vi "nanocal -- nuclear schottky fit V8.vi"() -> ()   [LabVIEW 2021] (continued)
 ,  \"στS\" -> 0.000000000000   ,  \"στN\" -> 0.000000000000   ,  \"τ11 \" -> 0.000000000000   ,  \"τ12\" -> 0.000000000000   ,  \"τ22\" -> 0.000000000000   ,  \"τN1\" -> 0.000000000000   ,  \"τN2\" -> 0.000000000000   ,  \"σηlogτ1 \" -> 0.000000000000   ,  \"σηlogτS\" -> 0.000000000000   ,  \"σηlogτN\" -> 0.000000000000   ,  \"σlogτ1\" -> 0.000000000000   ,  \"σlogτS\" -> 0.000000000000   ,  \"σlogτN\" -> 0.000000000000   ,  \"σητ1\" -> 0.000000000000   ,  \"σητS \" -> 0.000000000000   ,  \"σητN\" -> 0.000000000000    |>   , \r\"IDS0498_220603_RAW_cal__ref_\" ->   <|    \"ζ\" -> 0.110734162984   ,  \"τ1\" -> 0.019381596449   ,  \"τS\" -> 0.049800010244   ,  \"τN\" -> 0.007874153241   ,  \"τC\" -> 0.001094666009   ,  \"κ0\" -> 0.000000001580   ,  \"mm1\" -> 0.000107216591   ,  \"mm2\" -> 0.015930752272   ,  \"mm3\" -> 0.068498957299   ,  \"T\" -> 0.300000000000   ,  \"B\" -> 8.000000000000   ,  \"θ\" -> 45.000000000000   ,  \"Reoff\" -> -10657142.857142858200   ,  \"Imoff\" -> 0.000000000000   ,  \"στ1\" -> 0.007394501349   ,  \"στS\" -> 0.001744107422   ,  \"στN\" -> 0.001987690041   ,  \"τ11 \" -> 0.000000000000   ,  \"τ12\" -> 0.000000000000   ,  \"τ22\" -> 0.000000000000   ,  \"τN1\" -> 0.000000000000   ,  \"τN2\" -> 0.000000000000   ,  \"σηlogτ1 \" -> 0.000000000000   ,  \"σηlogτS\" -> 0.000000000000   ,  \"σηlogτN\" -> 0.000000000000   ,  \"σlogτ1\" -> 0.000000000000   ,  \"σlogτS\" -> 0.000000000000   ,  \"σlogτN\" -> 0.000000000000   ,  \"σητ1\" -> 0.000000000000   ,  \"σητS \" -> 0.000000000000   ,  \"σητN\" -> 0.000000000000    |>   , \r\"IDS0498_220603_RAW_cal__sam_\" ->   <|    \"ζ\" -> 0.000000000000   ,  \"τ1\" -> 0.000000000000   ,  \"τS\" -> 0.000000000000   ,  \"τN\" -> 0.000000000000   ,  \"τC\" -> 0.000000000000   ,  \"κ0\" -> 0.000000000000   ,  \"mm1\" -> 0.000000000000   ,  \"mm2\" -> 0.000000000000   ,  \"mm3\" -> 0.000000000000   ,  \"T\" -> 0.300000000000   ,  \"B\" -> 8.000000000000   ,  \"θ\" -> 45.000000000000   ,  \"Reoff\" -> 0.000000000000   ,  \"Imoff\" -> 0.000000000000   ,  \"στ1\" -> 0.000000000000   ,  \"στS\" -> 0.000000000000   ,  \"στN\" -> 0.000000000000   ,  \"τ11 \" -> 0.000000000000   ,  \"τ12\" -> 0.000000000000   ,  \"τ22\" -> 0.000000000000   ,  \"τN1\" -> 0.000000000000   ,  \"τN2\" -> 0.000000000000   ,  \"σηlogτ1 \" -> 0.000000000000   ,  \"σηlogτS\" -> 0.000000000000   ,  \"σηlogτN\" -> 0.000000000000   ,  \"σlogτ1\" -> 0.000000000000   ,  \"σlogτS\" -> 0.000000000000   ,  \"σlogτN\" -> 0.000000000000   ,  \"σητ1\" -> 0.000000000000   ,  \"σητS \" -> 0.000000000000   ,  \"σητN\" -> 0.000000000000    |>   , \r\"IDS0499_220603_RAW_cal__ref_\" ->   <|    \"ζ\" -> 0.075729964973   ,  \"τ1\" -> 0.017492157350   ,  \"τS\" -> 0.042916924435   ,  \"τN\" -> 0.003910009488   ,  \"τC\" -> 0.001485143735   ,  \"κ0\" -> 0.000000001996   ,  \"mm1\" -> 0.000101508308   ,  \"mm2\" -> 0.015465208626   ,  \"mm3\" -> 0.053783720140   ,  \"T\" -> 0.360000000000   ,  \"B\" -> 8.000000000000   ,  \"θ\" -> 45.000000000000   ,  \"Reoff\" -> -3787755.102040812380   ,  \"Imoff\" -> 0.000000000000   ,  \"στ1\" -> 0.001180089795   ,  \"στS\" -> 0.000447730504   ,  \"στN\" -> 0.000150733035   ,  \"τ11 \" -> 0.000000000000   ,  \"τ12\" -> 0.000000000000   ,  \"τ22\" -> 0.000000000000   ,  \"τN1\" -> 0.000000000000   ,  \"τN2\" -> 0.000000000000   ,  \"σηlogτ1 \" -> 0.000000000000   ,  \"σηlogτS\" -> 0.000000000000   ,  \"σηlogτN\" -> 0.000000000000   ,  \"σlogτ1\" -> 0.000000000000   ,  \"σlogτS\" -> 0.000000000000   ,  \"σlogτN\" -> 0.000000000000   ,  \"σητ1\" -> 0.000000000000   ,  \"σητS \" -> 0.000000000000   ,  \"σητN\" -> 0.000000000000    |>   , \r\"IDS0499_220603_RAW_cal__sam_\" ->   <|    \"ζ\" -> 0.000000000000   ,  \"τ1\" -> 0.000000000000   ,  \"τS\" -> 0.000000000000   ,  \"τN\" -> 0.000000000000   ,  \"τC\" -> 0.000000000000   ,  \"κ0\" -> 0.000000000000   ,  \"mm1\" -> 0.000000000000   ,  \"mm2\" -> 0.000000000000   ,  \"mm3\" -> 0.000000000000   ,  \"T\" -> 0.360000000000   ,  \"B\" -> 8.000000000000   ,  \"θ\" -> 45.000000000000   ,  \"Reoff\" -> 0.000000000000   ,  \"Imoff\" -> 0.000000000000   ,  \"στ1\" -> 0.000000000000   ,  \"στS\" -> 0.000000000000   ,  \"στN\" -> 0.000000000000   ,  \"τ11 \" -> 0.000000000000   ,  \"τ12\" -> 0.000000000000   ,  \"τ22\" -> 0.000000000000   ,  \"τN1\" -> 0.000000000000   ,  \"τN2\" -> 0.000000000000   ,  \"σηlogτ1 \" -> 0.000000000000   ,  \"σηlogτS\" -> 0.000000000000   ,  \"σηlogτN\" -> 0.000000000000   ,  \"σlogτ1\" -> 0.000000000000   ,  \"σlogτS\" -> 0.000000000000   ,  \"σlogτN\" -> 0.000000000000   ,  \"σητ1\" -> 0.000000000000   ,  \"σητS \" -> 0.000000000000   ,  \"σητN\" -> 0.000000000000    |>   , \r\"IDS0500_220603_RAW_cal__ref_\" ->   <|    \"ζ\" -> 0.057062025730   ,  \"τ1\" -> 0.015621328716   ,  \"τS\" -> 0.037684759429   ,  \"τN\" -> 0.002528358408   ,  \"τC\" -> 0.001814587656   ,  \"κ0\" -> 0.000000002409   ,  \"mm1\" -> 0.000093897005   ,  \"mm2\" -> 0.014229954054   ,  \"mm3\" -> 0.045619825114   ,  \"T\" -> 0.420000000000   ,  \"B\" -> 8.000000000000   ,  \"θ\" -> 45.000000000000   ,  \"Reoff\" -> -1914285.714285716420   ,  \"Imoff\" -> 0.000000000000   ,  \"στ1\" -> 0.000955516526   ,  \"στS\" -> 0.000234895501   ,  \"στN\" -> 0.000135281330   ,  \"τ11 \" -> 0.000000000000   ,  \"τ12\" -> 0.000000000000   ,  \"τ22\" -> 0.000000000000   ,  \"τN1\" -> 0.000000000000   ,  \"τN2\" -> 0.000000000000   ,  \"σηlogτ1 \" -> 0.000000000000   ,  \"σηlogτS\" -> 0.000000000000   ,  \"σηlogτN\" -> 0.000000000000   ,  \"σlogτ1\" -> 0.000000000000   ,  \"σlogτS\" -> 0.000000000000   ,  \"σlogτN\" -> 0.000000000000   ,  \"σητ1\" -> 0.000000000000   ,  \"σητS \" -> 0.000000000000   ,  \"σητN\" -> 0.000000000000    |>   , \r\"IDS0500_220603_RAW_cal__sam_\" ->   <|    \"ζ\" -> 0.000000000000   ,  \"τ1\" -> 0.000000000000   ,  \"τS\" -> 0.000000000000   ,  \"τN\" -> 0.000000000000   ,  \"τC\" -> 0.000000000000   ,  \"κ0\" -> 0.000000000000   ,  \"mm1\" -> 0.000000000000   ,  \"mm2\" -> 0.000000000000   ,  \"mm3\" -> 0.000000000000   ,  \"T\" -> 0.420000000000   ,  \"B\" -> 8.000000000000   ,  \"θ\" -> 45.000000000000   ,  \"Reoff\" -> 0.000000000000   ,  \"Imoff\" -> 0.000000000000   ,  \"στ1\" -> 0.000000000000   ,  \"στS\" -> 0.000000000000   ,  \"στN\" -> 0.000000000000   ,  \"τ11 \" -> 0.000000000000   ,  \"τ12\" -> 0.000000000000   ,  \"τ22\" -> 0.000000000000   ,  \"τN1\" -> 0.000000000000   ,  \"τN2\" -> 0.000000000000   ,  \"σηlogτ1 \" -> 0.000000000000   ,  \"σηlogτS\" -> 0.000000000000   ,  \"σηlogτN\" -> 0.000000000000   ,  \"σlogτ1\" -> 0.000000000000   ,  \"σlogτS\" -> 0.000000000000   ,  \"σlogτN\" -> 0.000000000000   ,  \"σητ1\" -> 0.000000000000   ,  \"σητS \" -> 0.000000000000   ,  \"σητN\" -> 0.000000000000    |>   , \r\"IDS0501_220603_RAW_cal__ref_\" ->   <|    \"ζ\" -> 0.041820610943   ,  \"τ1\" -> 0.014727705147   ,  \"τS\" -> 0.032103066270   ,  \"τN\" -> 0.001402697929   ,  \"τC\" -> 0.002062288671   ,  \"κ0\" -> 0.000000003070   ,  \"mm1\" -> 0.000078146988   ,  \"mm2\" -> 0.013796091461   ,  \"mm3\" -> 0.037822751096   ,  \"T\" -> 0.520000000000   ,  \"B\" -> 8.000000000000   ,  \"θ\" -> 45.000000000000   ,  \"Reoff\" -> -1155102.040816326160   ,  \"Imoff\" -> 0.000000000000   ,  \"στ1\" -> 0.000294282186   ,  \"στS\" -> 0.000104705305   ,  \"στN\" -> 0.000024302938   ,  \"τ11 \" -> 0.000000000000   ,  \"τ12\" -> 0.000000000000   ,  \"τ22\" -> 0.000000000000   ,  \"τN1\" -> 0.000000000000   ,  \"τN2\" -> 0.000000000000   ,  \"σηlogτ1 \" -> 0.000000000000   ,  \"σηlogτS\" -> 0.000000000000   ,  \"σηlogτN\" -> 0.000000000000   ,  \"σlogτ1\" -> 0.000000000000   ,  \"σlogτS\" -> 0.000000000000   ,  \"σlogτN\" -> 0.000000000000   ,  \"σητ1\" -> 0.000000000000   ,  \"σητS \" -> 0.000000000000   ,  \"σητN\" -> 0.000000000000    |>   , \r\"IDS0501_220603_RAW_cal__sam_\" ->   <|    \"ζ\" -> 0.000000000000   ,  \"τ1\" -> 0.000000000000   ,  \"τS\" -> 0.000000000000   ,  \"τN\" -> 0.000000000000   ,  \"τC\" -> 0.000000000000   ,  \"κ0\" -> 0.000000000000   ,  \"mm1\" -> 0.000000000000   ,  \"mm2\" -> 0.000000000000   ,  \"mm3\" -> 0.000000000000   ,  \"T\" -> 0.520000000000   ,  \"B\" -> 8.000000000000   ,  \"θ\" -> 45.000000000000   ,  \"Reoff\" -> 0.000000000000   ,  \"Imoff\" -> 0.000000000000   ,  \"στ1\" -> 0.000000000000   ,  \"στS\" -> 0.000000000000   ,  \"στN\" -> 0.000000000000   ,  \"τ11 \" -> 0.000000000000   ,  \"τ12\" -> 0.000000000000   ,  \"τ22\" -> 0.000000000000   ,  \"τN1\" -> 0.000000000000   ,  \"τN2\" -> 0.000000000000   ,  \"σηlogτ1 \" -> 0.000000000000   ,  \"σηlogτS\" -> 0.000000000000   ,  \"σηlogτN\" -> 0.000000000000   ,  \"σlogτ1\" -> 0.000000000000   ,  \"σlogτS\" -> 0.000000000000   ,  \"σlogτN\" -> 0.000000000000   ,  \"σητ1\" -> 0.000000000000   ,  \"σητS \" -> 0.000000000000   ,  \"σητN\" -> 0.000000000000    |>   , \r\"IDS0502_220603_RAW_cal__ref_\" ->   <|    \"ζ\" -> 0.034670986979   ,  \"τ1\" -> 0.014178027620   ,  \"τS\" -> 0.028243061757   ,  \"τN\" -> 0.000956770293   ,  \"τC\" -> 0.002118106957   ,  \"κ0\" -> 0.000000003766   ,  \"mm1\" -> 0.000066318852   ,  \"mm2\" -> 0.013432939767   ,  \"mm3\" -> 0.033009095005   ,  \"T\" -> 0.620000000000   ,  \"B\" -> 8.000000000000   ,  \"θ\" -> 45.000000000000   ,  \"Reoff\" -> -1228571.428571428170   ,  \"Imoff\" -> 0.000000000000   ,  \"στ1\" -> 0.000460475840   ,  \"στS\" -> 0.000103102463   ,  \"στN\" -> 0.000021520778   ,  \"τ11 \" -> 0.000000000000   ,  \"τ12\" -> 0.000000000000   ,  \"τ22\" -> 0.000000000000   ,  \"τN1\" -> 0.000000000000   ,  \"τN2\" -> 0.000000000000   ,  \"σηlogτ1 \" -> 0.000000000000   ,  \"σηlogτS\" -> 0.000000000000   ,  \"σηlogτN\" -> 0.000000000000   ,  \"σlogτ1\" -> 0.000000000000   ,  \"σlogτS\" -> 0.000000000000   ,  \"σlogτN\" -> 0.000000000000   ,  \"σητ1\" -> 0.000000000000   ,  \"σητS \" -> 0.000000000000   ,  \"σητN\" -> 0.000000000000    |>   , \r\"IDS0502_220603_RAW_cal__sam_\" ->   <|    \"ζ\" -> 0.000000000000   ,  \"τ1\" -> 0.000000000000   ,  \"τS\" -> 0.000000000000   ,  \"τN\" -> 0.000000000000   ,  \"τC\" -> 0.000000000000   ,  \"κ0\" -> 0.000000000000   ,  \"mm1\" -> 0.000000000000   ,  \"mm2\" -> 0.000000000000   ,  \"mm3\" -> 0.000000000000   ,  \"T\" -> 0.620000000000   ,  \"B\" -> 8.000000000000   ,  \"θ\" -> 45.000000000000   ,  \"Reoff\" -> 0.000000000000   ,  \"Imoff\" -> 0.000000000000   ,  \"στ1\" -> 0.000000000000   ,  \"στS\" -> 0.000000000000   ,  \"στN\" -> 0.000000000000   ,  \"τ11 \" -> 0.000000000000   ,  \"τ12\" -> 0.000000000000   ,  \"τ22\" -> 0.000000000000   ,  \"τN1\" -> 0.000000000000   ,  \"τN2\" -> 0.000000000000   ,  \"σηlogτ1 \" -> 0.000000000000   ,  \"σηlogτS\" -> 0.000000000000   ,  \"σηlogτN\" -> 0.000000000000   ,  \"σlogτ1\" -> 0.000000000000   ,  \"σlogτS\" -> 0.000000000000   ,  \"σlogτN\" -> 0.000000000000   ,  \"σητ1\" -> 0.000000000000   ,  \"σητS \" -> 0.000000000000   ,  \"σητN\" -> 0.000000000000    |>   , \r\"IDS0503_220603_RAW_cal__ref_\" ->   <|    \"ζ\" -> 0.027095379561   ,  \"τ1\" -> 0.013653054815   ,  \"τS\" -> 0.022995805893   ,  \"τN\" -> 0.000345510729   ,  \"τC\" -> 0.002402226581   ,  \"κ0\" -> 0.000000005139   ,  \"mm1\" -> 0.000057649125   ,  \"mm2\" -> 0.013281563049   ,  \"mm3\" -> 0.026689827678   ,  \"T\" -> 0.820000000000   ,  \"B\" -> 8.000000000000   ,  \"θ\" -> 45.000000000000   ,  \"Reoff\" -> -959183.673469387459   ,  \"Imoff\" -> 0.000000000000   ,  \"στ1\" -> 0.008451198848   ,  \"στS\" -> 0.000084348723   ,  \"στN\" -> 0.004631417027   ,  \"τ11 \" -> 0.000000000000   ,  \"τ12\" -> 0.000000000000   ,  \"τ22\" -> 0.000000000000   ,  \"τN1\" -> 0.000000000000   ,  \"τN2\" -> 0.000000000000   ,  \"σηlogτ1 \" -> 0.000000000000   ,  \"σηlogτS\" -> 0.000000000000   ,  \"σηlogτN\" -> 0.000000000000   ,  \"σlogτ1\" -> 0.000000000000   ,  \"σlogτS\" -> 0.000000000000   ,  \"σlogτN\" -> 0.000000000000   ,  \"σητ1\" -> 0.000000000000   ,  \"σητS \" -> 0.000000000000   ,  \"σητN\" -> 0.000000000000    |>   , \r\"IDS0503_220603_RAW_cal__sam_\" ->   <|    \"ζ\" -> 0.000000000000   ,  \"τ1\" -> 0.000000000000   ,  \"τS\" -> 0.000000000000   ,  \"τN\" -> 0.000000000000   ,  \"τC\" -> 0.000000000000   ,  \"κ0\" -> 0.000000000000   ,  \"mm1\" -> 0.000000000000   ,  \"mm2\" -> 0.000000000000   ,  \"mm3\" -> 0.000000000000   ,  \"T\" -> 0.820000000000   ,  \"B\" -> 8.000000000000   ,  \"θ\" -> 45.000000000000   ,  \"Reoff\" -> 0.000000000000   ,  \"Imoff\" -> 0.000000000000   ,  \"στ1\" -> 0.000000000000   ,  \"στS\" -> 0.000000000000   ,  \"στN\" -> 0.000000000000   ,  \"τ11 \" -> 0.000000000000   ,  \"τ12\" -> 0.000000000000   ,  \"τ22\" -> 0.000000000000   ,  \"τN1\" -> 0.000000000000   ,  \"τN2\" -> 0.000000000000   ,  \"σηlogτ1 \" -> 0.000000000000   ,  \"σηlogτS\" -> 0.000000000000   ,  \"σηlogτN\" -> 0.000000000000   ,  \"σlogτ1\" -> 0.000000000000   ,  \"σlogτS\" -> 0.000000000000   ,  \"σlogτN\" -> 0.000000000000   ,  \"σητ1\" -> 0.000000000000   ,  \"σητS \" -> 0.000000000000   ,  \"σητN\" -> 0.000000000000    |>   , \r\"IDS0504_220603_RAW_cal__ref_\" ->   <|    \"ζ\" -> 0.022447798358   ,  \"τ1\" -> 0.013732237823   ,  \"τS\" -> 0.018577417913   ,  \"τN\" -> 0.000137993980   ,  \"τC\" -> 0.002459582749   ,  \"κ0\" -> 0.000000007201   ,  \"mm1\" -> 0.000047916113   ,  \"mm2\" -> 0.013491821681   ,  \"mm3\" -> 0.021787614463   ,  \"T\" -> 1.120000000000   ,  \"B\" -> 8.000000000000   ,  \"θ\" -> 45.000000000000   ,  \"Reoff\" -> -714285.714285713619   ,  \"Imoff\" -> 0.000000000000   ,  \"στ1\" -> 0.022424406509   ,  \"στS\" -> 0.000101728053   ,  \"στN\" -> 0.011081871918   ,  \"τ11 \" -> 0.000000000000   ,  \"τ12\" -> 0.000000000000   ,  \"τ22\" -> 0.000000000000   ,  \"τN1\" -> 0.000000000000   ,  \"τN2\" -> 0.000000000000   ,  \"σηlogτ1 \" -> 0.000000000000   ,  \"σηlogτS\" -> 0.000000000000   ,  \"σηlogτN\" -> 0.000000000000   ,  \"σlogτ1\" -> 0.000000000000   ,  \"σlogτS\" -> 0.000000000000   ,  \"σlogτN\" -> 0.000000000000   ,  \"σητ1\" -> 0.000000000000   ,  \"σητS \" -> 0.000000000000   ,  \"σητN\" -> 0.000000000000    |>   , \r\"IDS0504_220603_RAW_cal__sam_\" ->   <|    \"ζ\" -> 0.000000000000   ,  \"τ1\" -> 0.000000000000   ,  \"τS\" -> 0.000000000000   ,  \"τN\" -> 0.000000000000   ,  \"τC\" -> 0.000000000000   ,  \"κ0\" -> 0.000000000000   ,  \"mm1\" -> 0.000000000000   ,  \"mm2\" -> 0.000000000000   ,  \"mm3\" -> 0.000000000000   ,  \"T\" -> 1.120000000000   ,  \"B\" -> 8.000000000000   ,  \"θ\" -> 45.000000000000   ,  \"Reoff\" -> 0.000000000000   ,  \"Imoff\" -> 0.000000000000   ,  \"στ1\" -> 0.000000000000   ,  \"στS\" -> 0.000000000000   ,  \"στN\" -> 0.000000000000   ,  \"τ11 \" -> 0.000000000000   ,  \"τ12\" -> 0.000000000000   ,  \"τ22\" -> 0.000000000000   ,  \"τN1\" -> 0.000000000000   ,  \"τN2\" -> 0.000000000000   ,  \"σηlogτ1 \" -> 0.000000000000   ,  \"σηlogτS\" -> 0.000000000000   ,  \"σηlogτN\" -> 0.000000000000   ,  \"σlogτ1\" -> 0.000000000000   ,  \"σlogτS\" -> 0.000000000000   ,  \"σlogτN\" -> 0.000000000000   ,  \"σητ1\" -> 0.000000000000   ,  \"σητS \" -> 0.000000000000   ,  \"σητN\" -> 0.000000000000    |>   , \r\"IDS0505_220603_RAW_cal__ref_\" ->   <|    \"ζ\" -> 0.017603951649   ,  \"τ1\" -> 0.013742471601   ,  \"τS\" -> 0.012869162108   ,  \"τN\" -> 0.000030445804   ,  \"τC\" -> 0.002783258647   ,  \"κ0\" -> 0.000000012669   ,  \"mm1\" -> 0.000039809007   ,  \"mm2\" -> 0.013558407618   ,  \"mm3\" -> 0.016054205609   ,  \"T\" -> 1.900000000000   ,  \"B\" -> 8.000000000000   ,  \"θ\" -> 45.000000000000   ,  \"Reoff\" -> -322448.979591836221   ,  \"Imoff\" -> 0.000000000000   ,  \"στ1\" -> 0.123558852950   ,  \"στS\" -> 0.000153637870   ,  \"στN\" -> 0.054392603462   ,  \"τ11 \" -> 0.000000000000   ,  \"τ12\" -> 0.000000000000   ,  \"τ22\" -> 0.000000000000   ,  \"τN1\" -> 0.000000000000   ,  \"τN2\" -> 0.000000000000   ,  \"σηlogτ1 \" -> 0.000000000000   ,  \"σηlogτS\" -> 0.000000000000   ,  \"σηlogτN\" -> 0.000000000000   ,  \"σlogτ1\" -> 0.000000000000   ,  \"σlogτS\" -> 0.000000000000   ,  \"σlogτN\" -> 0.000000000000   ,  \"σητ1\" -> 0.000000000000   ,  \"σητS \" -> 0.000000000000   ,  \"σητN\" -> 0.000000000000    |>   , \r\"IDS0505_220603_RAW_cal__sam_\" ->   <|    \"ζ\" -> 0.000000000000   ,  \"τ1\" -> 0.000000000000   ,  \"τS\" -> 0.000000000000   ,  \"τN\" -> 0.000000000000   ,  \"τC\" -> 0.000000000000   ,  \"κ0\" -> 0.000000000000   ,  \"mm1\" -> 0.000000000000   ,  \"mm2\" -> 0.000000000000   ,  \"mm3\" -> 0.000000000000   ,  \"T\" -> 1.900000000000   ,  \"B\" -> 8.000000000000   ,  \"θ\" -> 45.000000000000   ,  \"Reoff\" -> 0.000000000000   ,  \"Imoff\" -> 0.000000000000   ,  \"στ1\" -> 0.000000000000   ,  \"στS\" -> 0.000000000000   ,  \"στN\" -> 0.000000000000   ,  \"τ11 \" -> 0.000000000000   ,  \"τ12\" -> 0.000000000000   ,  \"τ22\" -> 0.000000000000   ,  \"τN1\" -> 0.000000000000   ,  \"τN2\" -> 0.000000000000   ,  \"σηlogτ1 \" -> 0.000000000000   ,  \"σηlogτS\" -> 0.000000000000   ,  \"σηlogτN\" -> 0.000000000000   ,  \"σlogτ1\" -> 0.000000000000   ,  \"σlogτS\" -> 0.000000000000   ,  \"σlogτN\" -> 0.000000000000   ,  \"σητ1\" -> 0.000000000000   ,  \"σητS \" -> 0.000000000000   ,  \"σητN\" -> 0.000000000000    |>   , \r\"IDS0506_220603_RAW_cal__ref_\" ->   <|    \"ζ\" -> 0.017513535650   ,  \"τ1\" -> 0.013742433942   ,  \"τS\" -> 0.009294247030   ,  \"τN\" -> 0.000005722768   ,  \"τC\" -> 0.002563999230   ,  \"κ0\" -> 0.000000022469   ,  \"mm1\" -> 0.000034819634   ,  \"mm2\" -> 0.011947473488   ,  \"mm3\" -> 0.013786985200   ,  \"T\" -> 3.100000000000   ,  \"B\" -> 8.000000000000   ,  \"θ\" -> 45.000000000000   ,  \"Reoff\" -> -175510.204081632197   ,  \"Imoff\" -> 0.000000000000   ,  \"στ1\" -> 0.880762480846   ,  \"στS\" -> 0.000241080362   ,  \"στN\" -> 0.387161662293   ,  \"τ11 \" -> 0.000000000000   ,  \"τ12\" -> 0.000000000000   ,  \"τ22\" -> 0.000000000000   ,  \"τN1\" -> 0.000000000000   ,  \"τN2\" -> 0.000000000000   ,  \"σηlogτ1 \" -> 0.000000000000   ,  \"σηlogτS\" -> 0.000000000000   ,  \"σηlogτN\" -> 0.000000000000   ,  \"σlogτ1\" -> 0.000000000000   ,  \"σlogτS\" -> 0.000000000000   ,  \"σlogτN\" -> 0.000000000000   ,  \"σητ1\" -> 0.000000000000   ,  \"σητS \" -> 0.000000000000   ,  \"σητN\" -> 0.000000000000    |>   , \r\"IDS0506_220603_RAW_cal__sam_\" ->   <|    \"ζ\" -> 0.000000000000   ,  \"τ1\" -> 0.000000000000   ,  \"τS\" -> 0.000000000000   ,  \"τN\" -> 0.000000000000   ,  \"τC\" -> 0.000000000000   ,  \"κ0\" -> 0.000000000000   ,  \"mm1\" -> 0.000000000000   ,  \"mm2\" -> 0.000000000000   ,  \"mm3\" -> 0.000000000000   ,  \"T\" -> 3.100000000000   ,  \"B\" -> 8.000000000000   ,  \"θ\" -> 45.000000000000   ,  \"Reoff\" -> 0.000000000000   ,  \"Imoff\" -> 0.000000000000   ,  \"στ1\" -> 0.000000000000   ,  \"στS\" -> 0.000000000000   ,  \"στN\" -> 0.000000000000   ,  \"τ11 \" -> 0.000000000000   ,  \"τ12\" -> 0.000000000000   ,  \"τ22\" -> 0.000000000000   ,  \"τN1\" -> 0.000000000000   ,  \"τN2\" -> 0.000000000000   ,  \"σηlogτ1 \" -> 0.000000000000   ,  \"σηlogτS\" -> 0.000000000000   ,  \"σηlogτN\" -> 0.000000000000   ,  \"σlogτ1\" -> 0.000000000000   ,  \"σlogτS\" -> 0.000000000000   ,  \"σlogτN\" -> 0.000000000000   ,  \"σητ1\" -> 0.000000000000   ,  \"σητS \" -> 0.000000000000   ,  \"σητN\" -> 0.000000000000    |>   , \r\"IDS0508_220603_RAW_cal__ref_\" ->   <|    \"ζ\" -> 0.243281471751   ,  \"τ1\" -> 0.025048654847   ,  \"τS\" -> 0.062611130643   ,  \"τN\" -> 0.020042988527   ,  \"τC\" -> 0.000849297815   ,  \"κ0\" -> 0.000000000907   ,  \"mm1\" -> 0.000164736185   ,  \"mm2\" -> 0.017764187201   ,  \"mm3\" -> 0.110731364203   ,  \"T\" -> 0.200000000000   ,  \"B\" -> 6.000000000000   ,  \"θ\" -> 45.000000000000   ,  \"Reoff\" -> -40636734.693877548000   ,  \"Imoff\" -> 0.000000000000   ,  \"στ1\" -> 0.014234353727   ,  \"στS\" -> 0.004838976210   ,  \"στN\" -> 0.004976250052   ,  \"τ11 \" -> 0.000000000000   ,  \"τ12\" -> 0.000000000000   ,  \"τ22\" -> 0.000000000000   ,  \"τN1\" -> 0.000000000000   ,  \"τN2\" -> 0.000000000000   ,  \"σηlogτ1 \" -> 0.000000000000   ,  \"σηlogτS\" -> 0.000000000000   ,  \"σηlogτN\" -> 0.000000000000   ,  \"σlogτ1\" -> 0.000000000000   ,  \"σlogτS\" -> 0.000000000000   ,  \"σlogτN\" -> 0.000000000000   ,  \"σητ1\" -> 0.000000000000   ,  \"σητS \" -> 0.000000000000   ,  \"σητN\" -> 0.000000000000    |>   , \r\"IDS0508_220603_RAW_cal__sam_\" ->   <|    \"ζ\" -> 0.000000000000   ,  \"τ1\" -> 0.000000000000   ,  \"τS\" -> 0.000000000000   ,  \"τN\" -> 0.000000000000   ,  \"τC\" -> 0.000000000000   ,  \"κ0\" -> 0.000000000000   ,  \"mm1\" -> 0.000000000000   ,  \"mm2\" -> 0.000000000000   ,  \"mm3\" -> 0.000000000000   ,  \"T\" -> 0.200000000000   ,  \"B\" -> 6.000000000000   ,  \"θ\" -> 45.000000000000   ,  \"Reoff\" -> 0.000000000000   ,  \"Imoff\" -> 0.000000000000   ,  \"στ1\" -> 0.000000000000   ,  \"στS\" -> 0.000000000000   ,  \"στN\" -> 0.000000000000   ,  \"τ11 \" -> 0.000000000000   ,  \"τ12\" -> 0.000000000000   ,  \"τ22\" -> 0.000000000000   ,  \"τN1\" -> 0.000000000000   ,  \"τN2\" -> 0.000000000000   ,  \"σηlogτ1 \" -> 0.000000000000   ,  \"σηlogτS\" -> 0.000000000000   ,  \"σηlogτN\" -> 0.000000000000   ,  \"σlogτ1\" -> 0.000000000000   ,  \"σlogτS\" -> 0.000000000000   ,  \"σlogτN\" -> 0.000000000000   ,  \"σητ1\" -> 0.000000000000   ,  \"σητS \" -> 0.000000000000   ,  \"σητN\" -> 0.000000000000    |>   , \r\"IDS0509_220603_RAW_cal__ref_\" ->   <|    \"ζ\" -> 0.413507557358   ,  \"τ1\" -> 0.033675995603   ,  \"τS\" -> 0.093816108912   ,  \"τN\" -> 0.061390510422   ,  \"τC\" -> 0.000803159189   ,  \"κ0\" -> 0.000000000612   ,  \"mm1\" -> 0.000233947412   ,  \"mm2\" -> 0.019125451380   ,  \"mm3\" -> 0.234505485381   ,  \"T\" -> 0.150000000000   ,  \"B\" -> 6.000000000000   ,  \"θ\" -> 45.000000000000   ,  \"Reoff\" -> -88975510.204081654600   ,  \"Imoff\" -> 0.000000000000   ,  \"στ1\" -> 0.030359635336   ,  \"στS\" -> 0.022777334435   ,  \"στN\" -> 0.025753606266   ,  \"τ11 \" -> 0.000000000000   ,  \"τ12\" -> 0.000000000000   ,  \"τ22\" -> 0.000000000000   ,  \"τN1\" -> 0.000000000000   ,  \"τN2\" -> 0.000000000000   ,  \"σηlogτ1 \" -> 0.000000000000   ,  \"σηlogτS\" -> 0.000000000000   ,  \"σηlogτN\" -> 0.000000000000   ,  \"σlogτ1\" -> 0.000000000000   ,  \"σlogτS\" -> 0.000000000000   ,  \"σlogτN\" -> 0.000000000000   ,  \"σητ1\" -> 0.000000000000   ,  \"σητS \" -> 0.000000000000   ,  \"σητN\" -> 0.000000000000    |>   , \r\"IDS0509_220603_RAW_cal__sam_\" ->   <|    \"ζ\" -> 0.000000000000   ,  \"τ1\" -> 0.000000000000   ,  \"τS\" -> 0.000000000000   ,  \"τN\" -> 0.000000000000   ,  \"τC\" -> 0.000000000000   ,  \"κ0\" -> 0.000000000000   ,  \"mm1\" -> 0.000000000000   ,  \"mm2\" -> 0.000000000000   ,  \"mm3\" -> 0.000000000000   ,  \"T\" -> 0.150000000000   ,  \"B\" -> 6.000000000000   ,  \"θ\" -> 45.000000000000   ,  \"Reoff\" -> 0.000000000000   ,  \"Imoff\" -> 0.000000000000   ,  \"στ1\" -> 0.000000000000   ,  \"στS\" -> 0.000000000000   ,  \"στN\" -> 0.000000000000   ,  \"τ11 \" -> 0.000000000000   ,  \"τ12\" -> 0.000000000000   ,  \"τ22\" -> 0.000000000000   ,  \"τN1\" -> 0.000000000000   ,  \"τN2\" -> 0.000000000000   ,  \"σηlogτ1 \" -> 0.000000000000   ,  \"σηlogτS\" -> 0.000000000000   ,  \"σηlogτN\" -> 0.000000000000   ,  \"σlogτ1\" -> 0.000000000000   ,  \"σlogτS\" -> 0.000000000000   ,  \"σlogτN\" -> 0.000000000000   ,  \"σητ1\" -> 0.000000000000   ,  \"σητS \" -> 0.000000000000   ,  \"σητN\" -> 0.000000000000    |>   , \r\"IDS0510_220603_RAW_cal__ref_\" ->   <|    \"ζ\" -> 0.613284276562   ,  \"τ1\" -> 0.039588841090   ,  \"τS\" -> 0.126363579952   ,  \"τN\" -> 0.150529821612   ,  \"τC\" -> 0.000834158039   ,  \"κ0\" -> 0.000000000449   ,  \"mm1\" -> 0.000316290952   ,  \"mm2\" -> 0.017230786632   ,  \"mm3\" -> 0.469583692571   ,  \"T\" -> 0.120000000000   ,  \"B\" -> 6.000000000000   ,  \"θ\" -> 45.000000000000   ,  \"Reoff\" -> -183040816.326530635000   ,  \"Imoff\" -> 0.000000000000   ,  \"στ1\" -> 0.058972518993   ,  \"στS\" -> 0.069910296081   ,  \"στN\" -> 0.097464298744   ,  \"τ11 \" -> 0.000000000000   ,  \"τ12\" -> 0.000000000000   ,  \"τ22\" -> 0.000000000000   ,  \"τN1\" -> 0.000000000000   ,  \"τN2\" -> 0.000000000000   ,  \"σηlogτ1 \" -> 0.000000000000   ,  \"σηlogτS\" -> 0.000000000000   ,  \"σηlogτN\" -> 0.000000000000   ,  \"σlogτ1\" -> 0.000000000000   ,  \"σlogτS\" -> 0.000000000000   ,  \"σlogτN\" -> 0.000000000000   ,  \"σητ1\" -> 0.000000000000   ,  \"σητS \" -> 0.000000000000   ,  \"σητN\" -> 0.000000000000    |>   , \r\"IDS0510_220603_RAW_cal__sam_\" ->   <|    \"ζ\" -> 0.000000000000   ,  \"τ1\" -> 0.000000000000   ,  \"τS\" -> 0.000000000000   ,  \"τN\" -> 0.000000000000   ,  \"τC\" -> 0.000000000000   ,  \"κ0\" -> 0.000000000000   ,  \"mm1\" -> 0.000000000000   ,  \"mm2\" -> 0.000000000000   ,  \"mm3\" -> 0.000000000000   ,  \"T\" -> 0.120000000000   ,  \"B\" -> 6.000000000000   ,  \"θ\" -> 45.000000000000   ,  \"Reoff\" -> 0.000000000000   ,  \"Imoff\" -> 0.000000000000   ,  \"στ1\" -> 0.000000000000   ,  \"στS\" -> 0.000000000000   ,  \"στN\" -> 0.000000000000   ,  \"τ11 \" -> 0.000000000000   ,  \"τ12\" -> 0.000000000000   ,  \"τ22\" -> 0.000000000000   ,  \"τN1\" -> 0.000000000000   ,  \"τN2\" -> 0.000000000000   ,  \"σηlogτ1 \" -> 0.000000000000   ,  \"σηlogτS\" -> 0.000000000000   ,  \"σηlogτN\" -> 0.000000000000   ,  \"σlogτ1\" -> 0.000000000000   ,  \"σlogτS\" -> 0.000000000000   ,  \"σlogτN\" -> 0.000000000000   ,  \"σητ1\" -> 0.000000000000   ,  \"σητS \" -> 0.000000000000   ,  \"σητN\" -> 0.000000000000    |>   , \r\"IDS0511_220604_RAW_cal__ref_\" ->   <|    \"ζ\" -> 0.330310083388   ,  \"τ1\" -> 0.030298910704   ,  \"τS\" -> 0.075236256272   ,  \"τN\" -> 0.040258490760   ,  \"τC\" -> 0.000782924983   ,  \"κ0\" -> 0.000000000728   ,  \"mm1\" -> 0.000193254303   ,  \"mm2\" -> 0.018356930637   ,  \"mm3\" -> 0.166175477301   ,  \"T\" -> 0.170000000000   ,  \"B\" -> 6.000000000000   ,  \"θ\" -> 45.000000000000   ,  \"Reoff\" -> -64436734.693877577800   ,  \"Imoff\" -> 0.000000000000   ,  \"στ1\" -> 0.014626951982   ,  \"στS\" -> 0.008056203133   ,  \"στN\" -> 0.008938953770   ,  \"τ11 \" -> 0.000000000000   ,  \"τ12\" -> 0.000000000000   ,  \"τ22\" -> 0.000000000000   ,  \"τN1\" -> 0.000000000000   ,  \"τN2\" -> 0.000000000000   ,  \"σηlogτ1 \" -> 0.000000000000   ,  \"σηlogτS\" -> 0.000000000000   ,  \"σηlogτN\" -> 0.000000000000   ,  \"σlogτ1\" -> 0.000000000000   ,  \"σlogτS\" -> 0.000000000000   ,  \"σlogτN\" -> 0.000000000000   ,  \"σητ1\" -> 0.000000000000   ,  \"σητS \" -> 0.000000000000   ,  \"σητN\" -> 0.000000000000    |>   , \r\"IDS0511_220604_RAW_cal__sam_\" ->   <|    \"ζ\" -> 0.000000000000   ,  \"τ1\" -> 0.000000000000   ,  \"τS\" -> 0.000000000000   ,  \"τN\" -> 0.000000000000   ,  \"τC\" -> 0.000000000000   ,  \"κ0\" -> 0.000000000000   ,  \"mm1\" -> 0.000000000000   ,  \"mm2\" -> 0.000000000000   ,  \"mm3\" -> 0.000000000000   ,  \"T\" -> 0.170000000000   ,  \"B\" -> 6.000000000000   ,  \"θ\" -> 45.000000000000   ,  \"Reoff\" -> 0.000000000000   ,  \"Imoff\" -> 0.000000000000   ,  \"στ1\" -> 0.000000000000   ,  \"στS\" -> 0.000000000000   ,  \"στN\" -> 0.000000000000   ,  \"τ11 \" -> 0.000000000000   ,  \"τ12\" -> 0.000000000000   ,  \"τ22\" -> 0.000000000000   ,  \"τN1\" -> 0.000000000000   ,  \"τN2\" -> 0.000000000000   ,  \"σηlogτ1 \" -> 0.000000000000   ,  \"σηlogτS\" -> 0.000000000000   ,  \"σηlogτN\" -> 0.000000000000   ,  \"σlogτ1\" -> 0.000000000000   ,  \"σlogτS\" -> 0.000000000000   ,  \"σlogτN\" -> 0.000000000000   ,  \"σητ1\" -> 0.000000000000   ,  \"σητS \" -> 0.000000000000   ,  \"σητN\" -> 0.000000000000    |>   , \r\"IDS0512_220604_RAW_cal__ref_\" ->   <|    \"ζ\" -> 0.157633362112   ,  \"τ1\" -> 0.020861334985   ,  \"τS\" -> 0.051508696686   ,  \"τN\" -> 0.008332770174   ,  \"τC\" -> 0.001009053466   ,  \"κ0\" -> 0.000000001248   ,  \"mm1\" -> 0.000135415312   ,  \"mm2\" -> 0.017070380875   ,  \"mm3\" -> 0.073939070739   ,  \"T\" -> 0.250000000000   ,  \"B\" -> 6.000000000000   ,  \"θ\" -> 45.000000000000   ,  \"Reoff\" -> -16726530.612244904000   ,  \"Imoff\" -> 0.000000000000   ,  \"στ1\" -> 0.019204175583   ,  \"στS\" -> 0.003261272874   ,  \"στN\" -> 0.003231373649   ,  \"τ11 \" -> 0.000000000000   ,  \"τ12\" -> 0.000000000000   ,  \"τ22\" -> 0.000000000000   ,  \"τN1\" -> 0.000000000000   ,  \"τN2\" -> 0.000000000000   ,  \"σηlogτ1 \" -> 0.000000000000   ,  \"σηlogτS\" -> 0.000000000000   ,  \"σηlogτN\" -> 0.000000000000   ,  \"σlogτ1\" -> 0.000000000000   ,  \"σlogτS\" -> 0.000000000000   ,  \"σlogτN\" -> 0.000000000000   ,  \"σητ1\" -> 0.000000000000   ,  \"σητS \" -> 0.000000000000   ,  \"σητN\" -> 0.000000000000    |>   , \r\"IDS0512_220604_RAW_cal__sam_\" ->   <|    \"ζ\" -> 0.000000000000   ,  \"τ1\" -> 0.000000000000   ,  \"τS\" -> 0.000000000000   ,  \"τN\" -> 0.000000000000   ,  \"τC\" -> 0.000000000000   ,  \"κ0\" -> 0.000000000000   ,  \"mm1\" -> 0.000000000000   ,  \"mm2\" -> 0.000000000000   ,  \"mm3\" -> 0.000000000000   ,  \"T\" -> 0.250000000000   ,  \"B\" -> 6.000000000000   ,  \"θ\" -> 45.000000000000   ,  \"Reoff\" -> 0.000000000000   ,  \"Imoff\" -> 0.000000000000   ,  \"στ1\" -> 0.000000000000   ,  \"στS\" -> 0.000000000000   ,  \"στN\" -> 0.000000000000   ,  \"τ11 \" -> 0.000000000000   ,  \"τ12\" -> 0.000000000000   ,  \"τ22\" -> 0.000000000000   ,  \"τN1\" -> 0.000000000000   ,  \"τN2\" -> 0.000000000000   ,  \"σηlogτ1 \" -> 0.000000000000   ,  \"σηlogτS\" -> 0.000000000000   ,  \"σηlogτN\" -> 0.000000000000   ,  \"σlogτ1\" -> 0.000000000000   ,  \"σlogτS\" -> 0.000000000000   ,  \"σlogτN\" -> 0.000000000000   ,  \"σητ1\" -> 0.000000000000   ,  \"σητS \" -> 0.000000000000   ,  \"σητN\" -> 0.000000000000    |>   , \r\"IDS0513_220604_RAW_cal__ref_\" ->   <|    \"ζ\" -> 0.109354643265   ,  \"τ1\" -> 0.019745794663   ,  \"τS\" -> 0.045929868636   ,  \"τN\" -> 0.004362632792   ,  \"τC\" -> 0.001089331798   ,  \"κ0\" -> 0.000000001568   ,  \"mm1\" -> 0.000105345441   ,  \"mm2\" -> 0.017323789537   ,  \"mm3\" -> 0.059198211464   ,  \"T\" -> 0.300000000000   ,  \"B\" -> 6.000000000000   ,  \"θ\" -> 45.000000000000   ,  \"Reoff\" -> -9718367.346938773990   ,  \"Imoff\" -> 0.000000000000   ,  \"στ1\" -> 0.000746121350   ,  \"στS\" -> 0.000145078797   ,  \"στN\" -> 0.000139513521   ,  \"τ11 \" -> 0.000000000000   ,  \"τ12\" -> 0.000000000000   ,  \"τ22\" -> 0.000000000000   ,  \"τN1\" -> 0.000000000000   ,  \"τN2\" -> 0.000000000000   ,  \"σηlogτ1 \" -> 0.000000000000   ,  \"σηlogτS\" -> 0.000000000000   ,  \"σηlogτN\" -> 0.000000000000   ,  \"σlogτ1\" -> 0.000000000000   ,  \"σlogτS\" -> 0.000000000000   ,  \"σlogτN\" -> 0.000000000000   ,  \"σητ1\" -> 0.000000000000   ,  \"σητS \" -> 0.000000000000   ,  \"σητN\" -> 0.000000000000    |>   , \r\"IDS0513_220604_RAW_cal__sam_\" ->   <|    \"ζ\" -> 0.000000000000   ,  \"τ1\" -> 0.000000000000   ,  \"τS\" -> 0.000000000000   ,  \"τN\" -> 0.000000000000   ,  \"τC\" -> 0.000000000000   ,  \"κ0\" -> 0.000000000000   ,  \"mm1\" -> 0.000000000000   ,  \"mm2\" -> 0.000000000000   ,  \"mm3\" -> 0.000000000000   ,  \"T\" -> 0.300000000000   ,  \"B\" -> 6.000000000000   ,  \"θ\" -> 45.000000000000   ,  \"Reoff\" -> 0.000000000000   ,  \"Imoff\" -> 0.000000000000   ,  \"στ1\" -> 0.000000000000   ,  \"στS\" -> 0.000000000000   ,  \"στN\" -> 0.000000000000   ,  \"τ11 \" -> 0.000000000000   ,  \"τ12\" -> 0.000000000000   ,  \"τ22\" -> 0.000000000000   ,  \"τN1\" -> 0.000000000000   ,  \"τN2\" -> 0.000000000000   ,  \"σηlogτ1 \" -> 0.000000000000   ,  \"σηlogτS\" -> 0.000000000000   ,  \"σηlogτN\" -> 0.000000000000   ,  \"σlogτ1\" -> 0.000000000000   ,  \"σlogτS\" -> 0.000000000000   ,  \"σlogτN\" -> 0.000000000000   ,  \"σητ1\" -> 0.000000000000   ,  \"σητS \" -> 0.000000000000   ,  \"σητN\" -> 0.000000000000    |>   , \r\"IDS0514_220604_RAW_cal__ref_\" ->   <|    \"ζ\" -> 0.078464971050   ,  \"τ1\" -> 0.017563831776   ,  \"τS\" -> 0.042315631100   ,  \"τN\" -> 0.002449698464   ,  \"τC\" -> 0.001311085354   ,  \"κ0\" -> 0.000000001978   ,  \"mm1\" -> 0.000092908726   ,  \"mm2\" -> 0.016171593309   ,  \"mm3\" -> 0.050888254947   ,  \"T\" -> 0.360000000000   ,  \"B\" -> 6.000000000000   ,  \"θ\" -> 45.000000000000   ,  \"Reoff\" -> -5555102.040816326630   ,  \"Imoff\" -> 0.000000000000   ,  \"στ1\" -> 0.001705710692   ,  \"στS\" -> 0.000224693737   ,  \"στN\" -> 0.000168766252   ,  \"τ11 \" -> 0.000000000000   ,  \"τ12\" -> 0.000000000000   ,  \"τ22\" -> 0.000000000000   ,  \"τN1\" -> 0.000000000000   ,  \"τN2\" -> 0.000000000000   ,  \"σηlogτ1 \" -> 0.000000000000   ,  \"σηlogτS\" -> 0.000000000000   ,  \"σηlogτN\" -> 0.000000000000   ,  \"σlogτ1\" -> 0.000000000000   ,  \"σlogτS\" -> 0.000000000000   ,  \"σlogτN\" -> 0.000000000000   ,  \"σητ1\" -> 0.000000000000   ,  \"σητS \" -> 0.000000000000   ,  \"σητN\" -> 0.000000000000    |>   , \r\"IDS0514_220604_RAW_cal__sam_\" ->   <|    \"ζ\" -> 0.000000000000   ,  \"τ1\" -> 0.000000000000   ,  \"τS\" -> 0.000000000000   ,  \"τN\" -> 0.000000000000   ,  \"τC\" -> 0.000000000000   ,  \"κ0\" -> 0.000000000000   ,  \"mm1\" -> 0.000000000000   ,  \"mm2\" -> 0.000000000000   ,  \"mm3\" -> 0.000000000000   ,  \"T\" -> 0.360000000000   ,  \"B\" -> 6.000000000000   ,  \"θ\" -> 45.000000000000   ,  \"Reoff\" -> 0.000000000000   ,  \"Imoff\" -> 0.000000000000   ,  \"στ1\" -> 0.000000000000   ,  \"στS\" -> 0.000000000000   ,  \"στN\" -> 0.000000000000   ,  \"τ11 \" -> 0.000000000000   ,  \"τ12\" -> 0.000000000000   ,  \"τ22\" -> 0.000000000000   ,  \"τN1\" -> 0.000000000000   ,  \"τN2\" -> 0.000000000000   ,  \"σηlogτ1 \" -> 0.000000000000   ,  \"σηlogτS\" -> 0.000000000000   ,  \"σηlogτN\" -> 0.000000000000   ,  \"σlogτ1\" -> 0.000000000000   ,  \"σlogτS\" -> 0.000000000000   ,  \"σlogτN\" -> 0.000000000000   ,  \"σητ1\" -> 0.000000000000   ,  \"σητS \" -> 0.000000000000   ,  \"σητN\" -> 0.000000000000    |>   , \r\"IDS0515_220604_RAW_cal__ref_\" ->   <|    \"ζ\" -> 0.061585995431   ,  \"τ1\" -> 0.017021907134   ,  \"τS\" -> 0.041190711561   ,  \"τN\" -> 0.001409585610   ,  \"τC\" -> 0.001428995669   ,  \"κ0\" -> 0.000000002390   ,  \"mm1\" -> 0.000080420011   ,  \"mm2\" -> 0.016183837088   ,  \"mm3\" -> 0.047410524581   ,  \"T\" -> 0.430000000000   ,  \"B\" -> 6.000000000000   ,  \"θ\" -> 45.000000000000   ,  \"Reoff\" -> -4253061.224489795980   ,  \"Imoff\" -> 0.000000000000   ,  \"στ1\" -> 0.002084861078   ,  \"στS\" -> 0.000053084466   ,  \"στN\" -> 0.001354478999   ,  \"τ11 \" -> 0.000000000000   ,  \"τ12\" -> 0.000000000000   ,  \"τ22\" -> 0.000000000000   ,  \"τN1\" -> 0.000000000000   ,  \"τN2\" -> 0.000000000000   ,  \"σηlogτ1 \" -> 0.000000000000   ,  \"σηlogτS\" -> 0.000000000000   ,  \"σηlogτN\" -> 0.000000000000   ,  \"σlogτ1\" -> 0.000000000000   ,  \"σlogτS\" -> 0.000000000000   ,  \"σlogτN\" -> 0.000000000000   ,  \"σητ1\" -> 0.000000000000   ,  \"σητS \" -> 0.000000000000   ,  \"σητN\" -> 0.000000000000    |>   , \r\"IDS0515_220604_RAW_cal__sam_\" ->   <|    \"ζ\" -> 0.000000000000   ,  \"τ1\" -> 0.000000000000   ,  \"τS\" -> 0.000000000000   ,  \"τN\" -> 0.000000000000   ,  \"τC\" -> 0.000000000000   ,  \"κ0\" -> 0.000000000000   ,  \"mm1\" -> 0.000000000000   ,  \"mm2\" -> 0.000000000000   ,  \"mm3\" -> 0.000000000000   ,  \"T\" -> 0.430000000000   ,  \"B\" -> 6.000000000000   ,  \"θ\" -> 45.000000000000   ,  \"Reoff\" -> 0.000000000000   ,  \"Imoff\" -> 0.000000000000   ,  \"στ1\" -> 0.000000000000   ,  \"στS\" -> 0.000000000000   ,  \"στN\" -> 0.000000000000   ,  \"τ11 \" -> 0.000000000000   ,  \"τ12\" -> 0.000000000000   ,  \"τ22\" -> 0.000000000000   ,  \"τN1\" -> 0.000000000000   ,  \"τN2\" -> 0.000000000000   ,  \"σηlogτ1 \" -> 0.000000000000   ,  \"σηlogτS\" -> 0.000000000000   ,  \"σηlogτN\" -> 0.000000000000   ,  \"σlogτ1\" -> 0.000000000000   ,  \"σlogτS\" -> 0.000000000000   ,  \"σlogτN\" -> 0.000000000000   ,  \"σητ1\" -> 0.000000000000   ,  \"σητS \" -> 0.000000000000   ,  \"σητN\" -> 0.000000000000    |>   , \r\"IDS0516_220604_RAW_cal__ref_\" ->   <|    \"ζ\" -> 0.045061124228   ,  \"τ1\" -> 0.016174333666   ,  \"τS\" -> 0.041331628225   ,  \"τN\" -> 0.000750592529   ,  \"τC\" -> 0.001666143406   ,  \"κ0\" -> 0.000000003072   ,  \"mm1\" -> 0.000069279623   ,  \"mm2\" -> 0.015749025797   ,  \"mm3\" -> 0.046000664583   ,  \"T\" -> 0.520000000000   ,  \"B\" -> 6.000000000000   ,  \"θ\" -> 45.000000000000   ,  \"Reoff\" -> -2636734.693877550770   ,  \"Imoff\" -> 0.000000000000   ,  \"στ1\" -> 0.005008431777   ,  \"στS\" -> 0.000068540084   ,  \"στN\" -> 0.003310443963   ,  \"τ11 \" -> 0.000000000000   ,  \"τ12\" -> 0.000000000000   ,  \"τ22\" -> 0.000000000000   ,  \"τN1\" -> 0.000000000000   ,  \"τN2\" -> 0.000000000000   ,  \"σηlogτ1 \" -> 0.000000000000   ,  \"σηlogτS\" -> 0.000000000000   ,  \"σηlogτN\" -> 0.000000000000   ,  \"σlogτ1\" -> 0.000000000000   ,  \"σlogτS\" -> 0.000000000000   ,  \"σlogτN\" -> 0.000000000000   ,  \"σητ1\" -> 0.000000000000   ,  \"σητS \" -> 0.000000000000   ,  \"σητN\" -> 0.000000000000    |>   , \r\"IDS0516_220604_RAW_cal__sam_\" ->   <|    \"ζ\" -> 0.000000000000   ,  \"τ1\" -> 0.000000000000   ,  \"τS\" -> 0.000000000000   ,  \"τN\" -> 0.000000000000   ,  \"τC\" -> 0.000000000000   ,  \"κ0\" -> 0.000000000000   ,  \"mm1\" -> 0.000000000000   ,  \"mm2\" -> 0.000000000000   ,  \"mm3\" -> 0.000000000000   ,  \"T\" -> 0.520000000000   ,  \"B\" -> 6.000000000000   ,  \"θ\" -> 45.000000000000   ,  \"Reoff\" -> 0.000000000000   ,  \"Imoff\" -> 0.000000000000   ,  \"στ1\" -> 0.000000000000   ,  \"στS\" -> 0.000000000000   ,  \"στN\" -> 0.000000000000   ,  \"τ11 \" -> 0.000000000000   ,  \"τ12\" -> 0.000000000000   ,  \"τ22\" -> 0.000000000000   ,  \"τN1\" -> 0.000000000000   ,  \"τN2\" -> 0.000000000000   ,  \"σηlogτ1 \" -> 0.000000000000   ,  \"σηlogτS\" -> 0.000000000000   ,  \"σηlogτN\" -> 0.000000000000   ,  \"σlogτ1\" -> 0.000000000000   ,  \"σlogτS\" -> 0.000000000000   ,  \"σlogτN\" -> 0.000000000000   ,  \"σητ1\" -> 0.000000000000   ,  \"σητS \" -> 0.000000000000   ,  \"σητN\" -> 0.000000000000    |>   , \r\"IDS0517_220604_RAW_cal__ref_\" ->   <|    \"ζ\" -> 0.037661249073   ,  \"τ1\" -> 0.016158267438   ,  \"τS\" -> 0.041535470501   ,  \"τN\" -> 0.000443947438   ,  \"τC\" -> 0.001574909889   ,  \"κ0\" -> 0.000000003727   ,  \"mm1\" -> 0.000055213447   ,  \"mm2\" -> 0.015903179567   ,  \"mm3\" -> 0.045335199567   ,  \"T\" -> 0.620000000000   ,  \"B\" -> 6.000000000000   ,  \"θ\" -> 45.000000000000   ,  \"Reoff\" -> -2277551.020408163780   ,  \"Imoff\" -> 0.000000000000   ,  \"στ1\" -> 0.010069463769   ,  \"στS\" -> 0.000081017666   ,  \"στN\" -> 0.006636828658   ,  \"τ11 \" -> 0.000000000000   ,  \"τ12\" -> 0.000000000000   ,  \"τ22\" -> 0.000000000000   ,  \"τN1\" -> 0.000000000000   ,  \"τN2\" -> 0.000000000000   ,  \"σηlogτ1 \" -> 0.000000000000   ,  \"σηlogτS\" -> 0.000000000000   ,  \"σηlogτN\" -> 0.000000000000   ,  \"σlogτ1\" -> 0.000000000000   ,  \"σlogτS\" -> 0.000000000000   ,  \"σlogτN\" -> 0.000000000000   ,  \"σητ1\" -> 0.000000000000   ,  \"σητS \" -> 0.000000000000   ,  \"σητN\" -> 0.000000000000    |>   , \r\"IDS0517_220604_RAW_cal__sam_\" ->   <|    \"ζ\" -> 0.000000000000   ,  \"τ1\" -> 0.000000000000   ,  \"τS\" -> 0.000000000000   ,  \"τN\" -> 0.000000000000   ,  \"τC\" -> 0.000000000000   ,  \"κ0\" -> 0.000000000000   ,  \"mm1\" -> 0.000000000000   ,  \"mm2\" -> 0.000000000000   ,  \"mm3\" -> 0.000000000000   ,  \"T\" -> 0.620000000000   ,  \"B\" -> 6.000000000000   ,  \"θ\" -> 45.000000000000   ,  \"Reoff\" -> 0.000000000000   ,  \"Imoff\" -> 0.000000000000   ,  \"στ1\" -> 0.000000000000   ,  \"στS\" -> 0.000000000000   ,  \"στN\" -> 0.000000000000   ,  \"τ11 \" -> 0.000000000000   ,  \"τ12\" -> 0.000000000000   ,  \"τ22\" -> 0.000000000000   ,  \"τN1\" -> 0.000000000000   ,  \"τN2\" -> 0.000000000000   ,  \"σηlogτ1 \" -> 0.000000000000   ,  \"σηlogτS\" -> 0.000000000000   ,  \"σηlogτN\" -> 0.000000000000   ,  \"σlogτ1\" -> 0.000000000000   ,  \"σlogτS\" -> 0.000000000000   ,  \"σlogτN\" -> 0.000000000000   ,  \"σητ1\" -> 0.000000000000   ,  \"σητS \" -> 0.000000000000   ,  \"σητN\" -> 0.000000000000    |>   , \r\"IDS0518_220604_RAW_cal__ref_\" ->   <|    \"ζ\" -> 0.026897195586   ,  \"τ1\" -> 0.017029322947   ,  \"τS\" -> 0.030300618121   ,  \"τN\" -> 0.000170844478   ,  
